vi "dynamic signal reproduction.vi"() -> ()   [LabVIEW 2016]
panel:
  in  "scaling ratio (zero for default)":dbl
  in  "Analog out":string(combo)
  out "X":dbl[](array[numeric])
  in  "X file path":path
  in  "rate":dbl
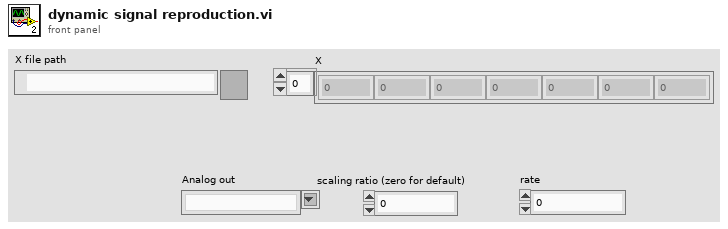
[diagram p1: front panel]
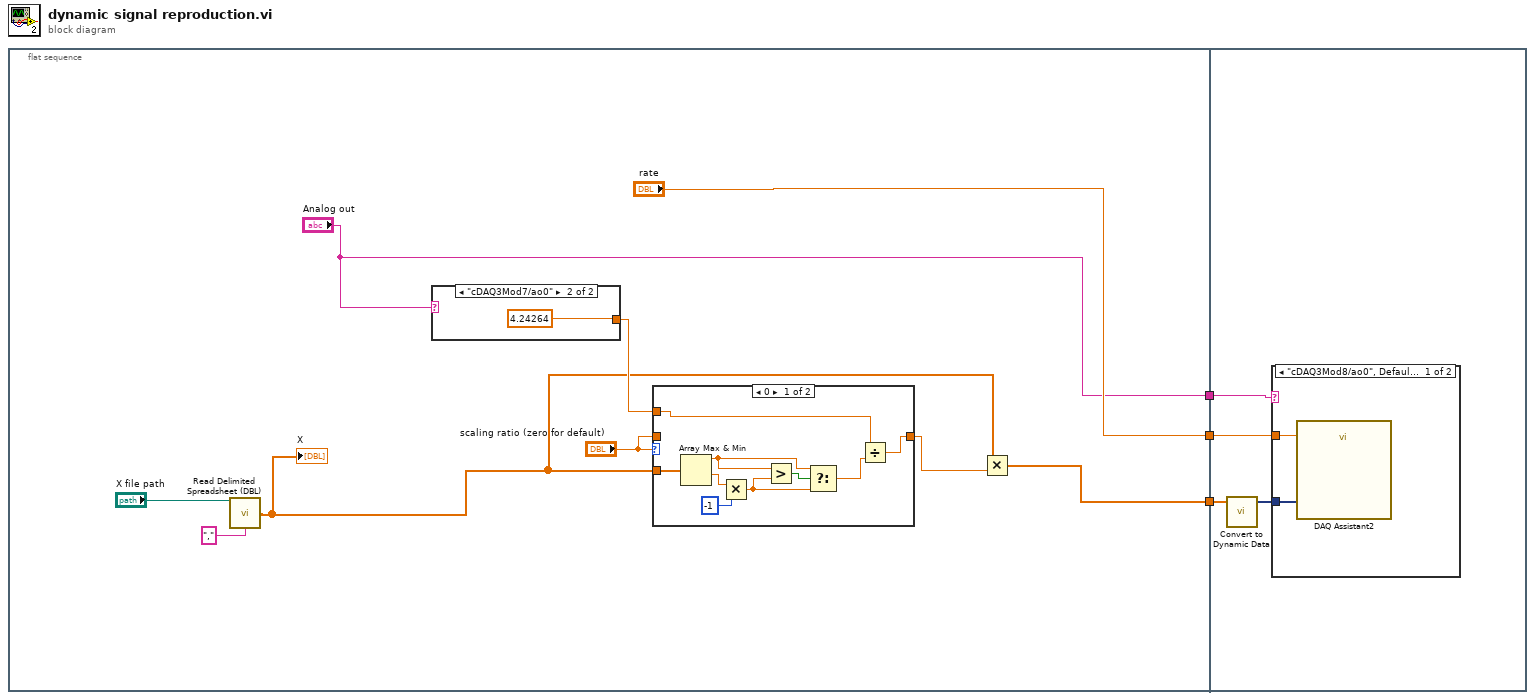
[diagram p0: block diagram]
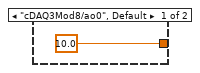
[diagram p2: hidden frame]
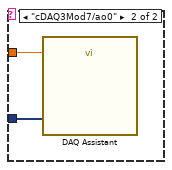
[diagram p4: hidden frame]
diagram:
  n1 = flat-sequence {
    tunnel: ["rate"] -> w3
    tunnel: [w7] -> w2
    tunnel: ["Analog out"] -> w1
    tunnel: w1 -> [w25]
    tunnel: w2 -> [w27]
    tunnel: w3 -> [w28]
    frame #0 {
      n2 = call <vilib>:"Read Delimited Spreadsheet (DBL).vi"("file path (dialog if empty)"="X file path", "delimiter (\\t)"=",") -> ("first row"=w5:dbl[])  [unwired: 8 in, 5 out]
      "X" <- w5
      n3 = case shown="\"cDAQ3Mod7/ao0\"" "Analog out" {
        tunnel: [10.0 4.24264] -> w9
        frame "cDAQ3Mod8/ao0", Default {
        }
        frame "cDAQ3Mod7/ao0" {
        }
      }
      n4 = case shown="0" "scaling ratio (zero for default)" {
        tunnel: w9 -> [w17 _]
        tunnel: "scaling ratio (zero for default)" -> [_ w24]
        tunnel: [w15 w24] -> w4
        tunnel: w5 -> [w18 _]
        frame 0 {
          n5 = Array Max & Min(array=w18) -> (max value=w21:dbl, min value=w20:dbl)  [unwired: 2 out]
          n6 = Multiply(x=w20, y=-1) -> (x*y=w22:dbl)
          n7 = Greater?(x=w21, y=w22) -> (0:w23:bool)
          n8 = Select(t=w21, s=w23, f=w22) -> (s? t:f=w16:dbl)
          n9 = Divide(x=w17, y=w16) -> (x/y=w15:dbl)
        }
        frame 1, Default {
        }
      }
      n10 = Multiply(x=w5, y=w4) -> (x*y=w7:dbl[])
    }
    frame #1 {
      n11 = call "Convert to Dynamic Data"("Array"=w27) -> ("Dynamic Data Type"=w26:dynamicdata)  [unwired: 3 in]
      n12 = case shown="\"cDAQ3Mod8/ao0\", Default" w25 {
        tunnel: w28 -> [w30 w32]
        tunnel: w26 -> [w29 w31]
        frame "cDAQ3Mod8/ao0", Default {
          n13 = call "DAQ Assistant2"("data"=w29, "rate"=w30) -> ()  [unwired: 15 in, 3 out]
        }
        frame "cDAQ3Mod7/ao0" {
          n14 = call "DAQ Assistant"("data"=w31, "rate"=w32) -> ()  [unwired: 15 in, 3 out]
        }
      }
    }
  }
